vi "Linecut.vi"() -> ()   [LabVIEW 2019]
uses:
  graph_utilities.lvclass
panel:
  out "x-y":dbl
  in  "OK":bool
  in  "width (horizontal) 2":dbl=0.2
  in  "width (vertical) 2":dbl=0.2
  out "Horizontal 2":cluster{dbl[], dbl[]}[](graph)
  out "Vertical 2":cluster{dbl[], dbl[]}[](graph)
  out "Target:":dbl[][](graph)
  in  "width (horizontal)":dbl=0.2
  in  "width (vertical)":dbl=0.2
  out "Horizontal":cluster{dbl[], dbl[]}[](graph)
  out "Vertical":cluster{dbl[], dbl[]}[](graph)
  out "Control:":dbl[][](graph)
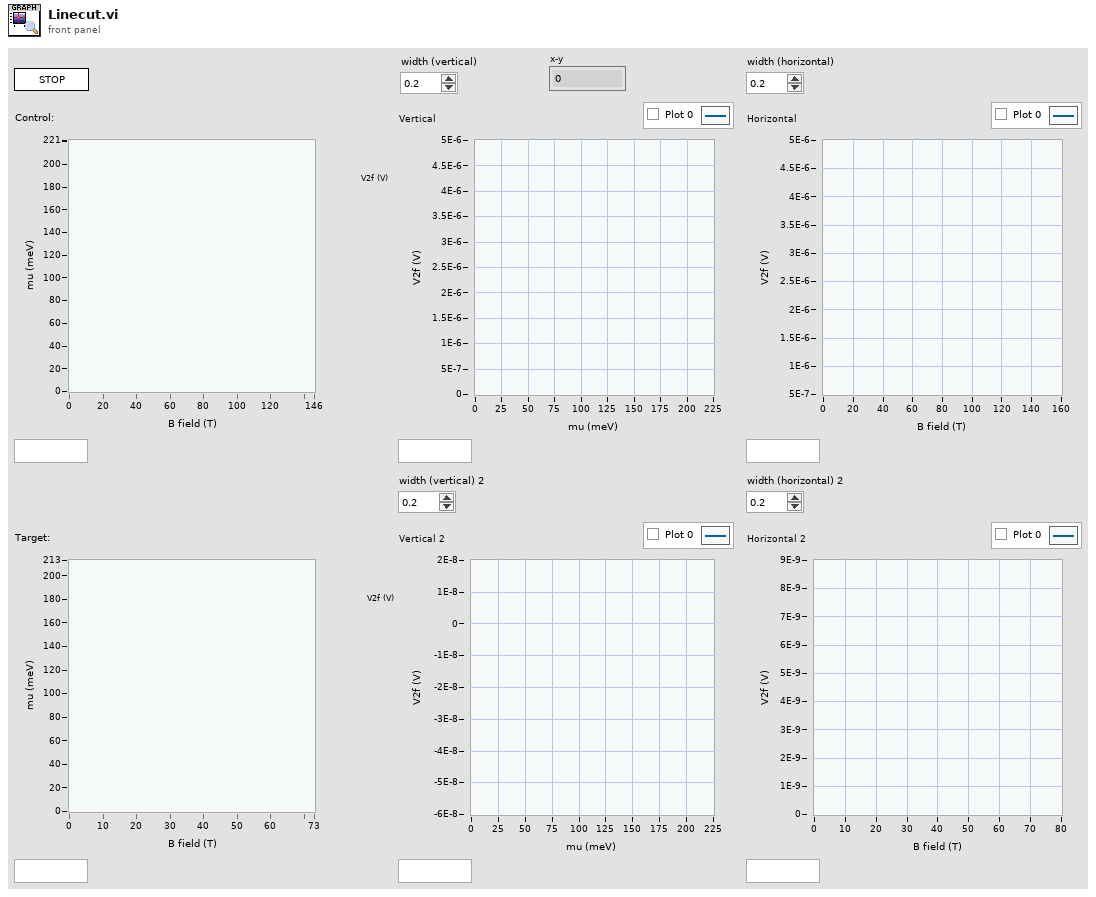
[diagram p1: front panel]
types:
  T1 = enum32{"Invalid", "Standard", "Closed", "Hidden", "Minimized", "Maximized"}
  T2 = enum32{"invalid app kind", "Development System", "Run Time System", "Student Edition", "Embedded LabVIEW", "Evaluation", "Custom"}
  T3 = cluster{"Core":cluster{"Current VI Reference":refnum<vi>, "Close Panel on Exit?":bool}, "graphs":refnum<class "graph_utilities.lvclass">[]}
  T4 = cluster{"Current VI Reference":refnum<vi>, "Close Panel on Exit?":bool}
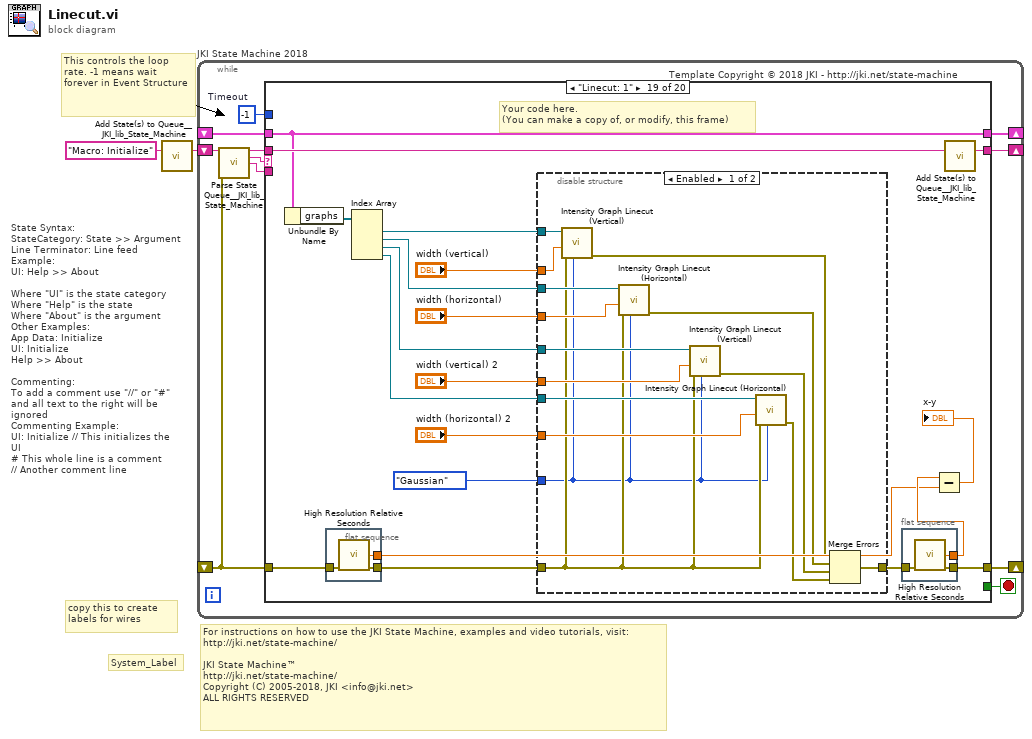
[diagram p0: block diagram]
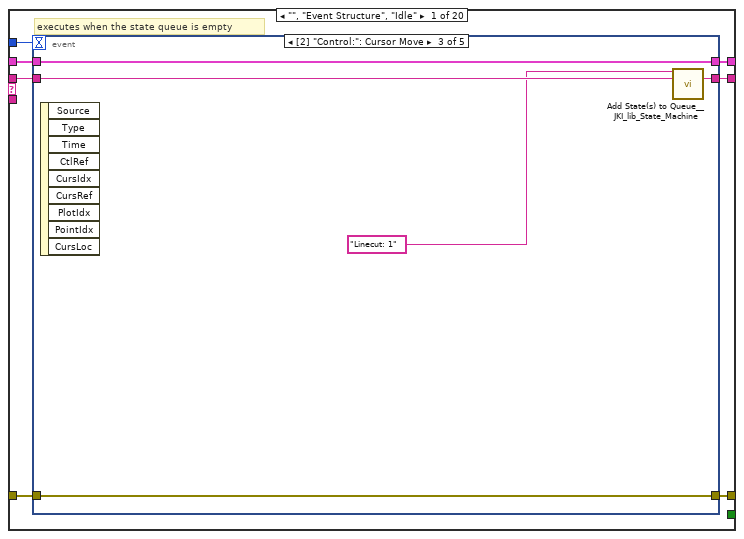
[diagram p2: hidden frame]
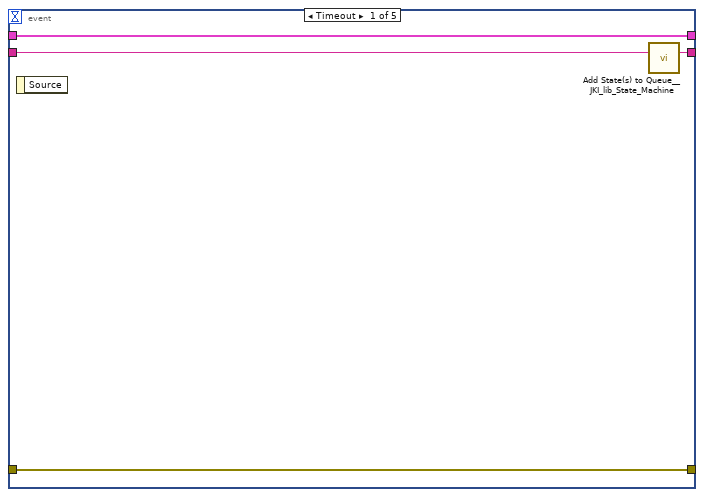
[diagram p3: hidden frame]
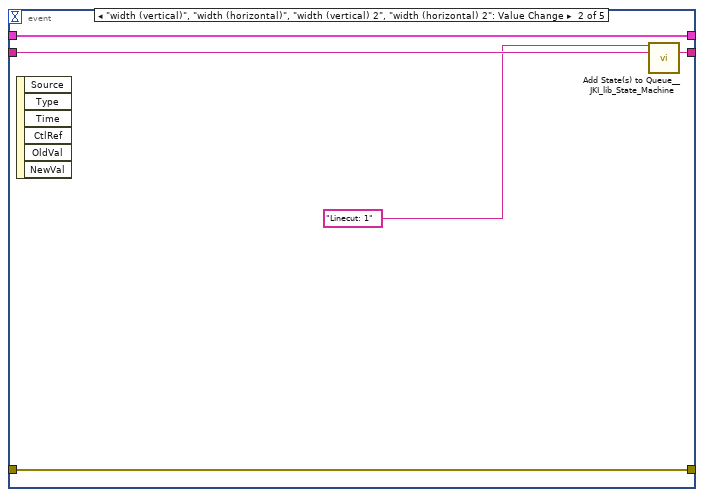
[diagram p4: hidden frame]
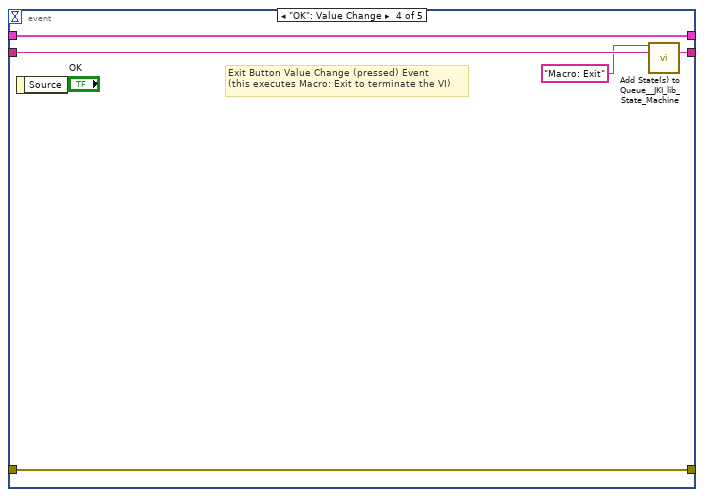
[diagram p5: hidden frame]
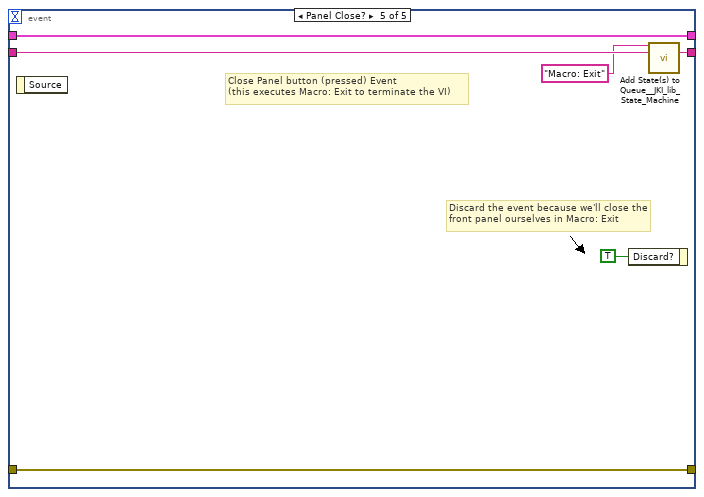
[diagram p6: hidden frame]
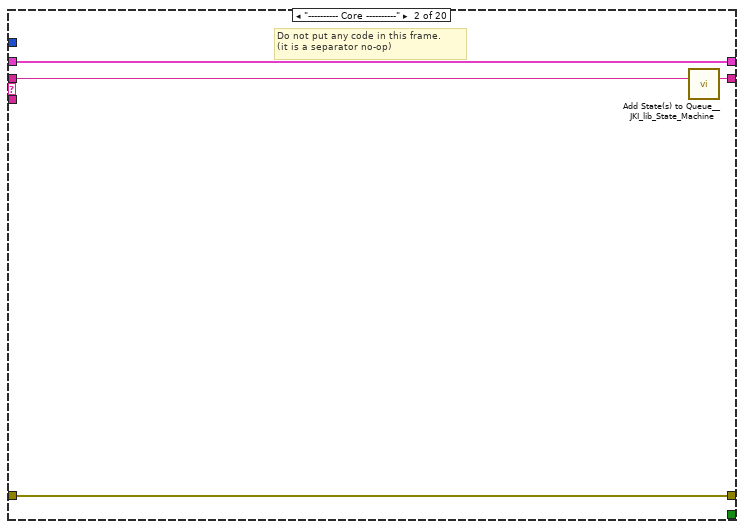
[diagram p7: hidden frame]
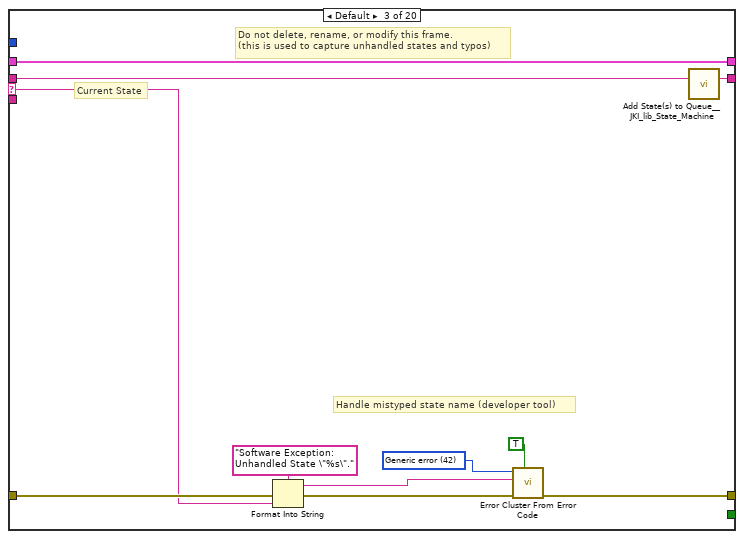
[diagram p8: hidden frame]
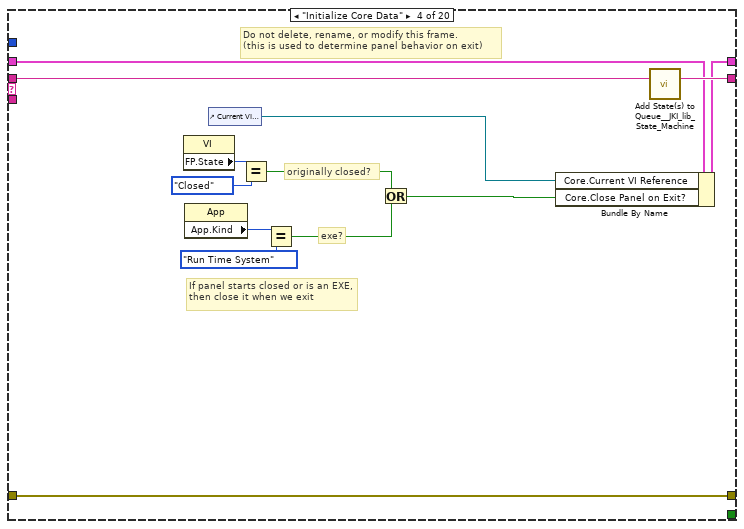
[diagram p9: hidden frame]
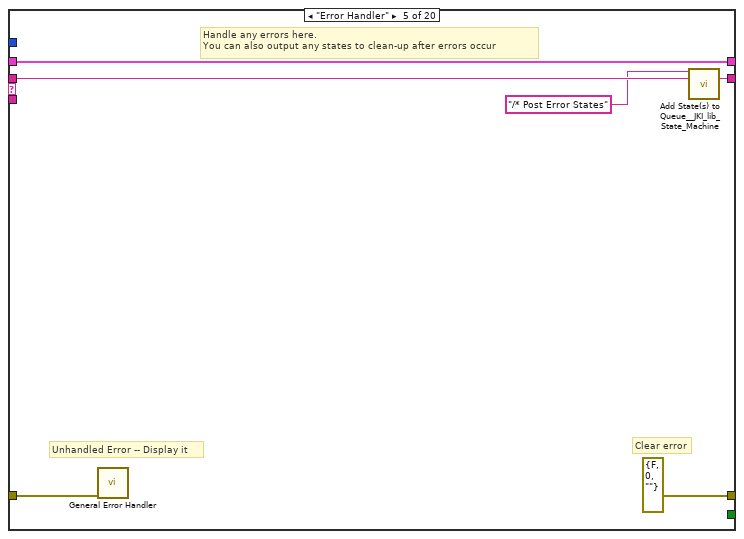
[diagram p10: hidden frame]
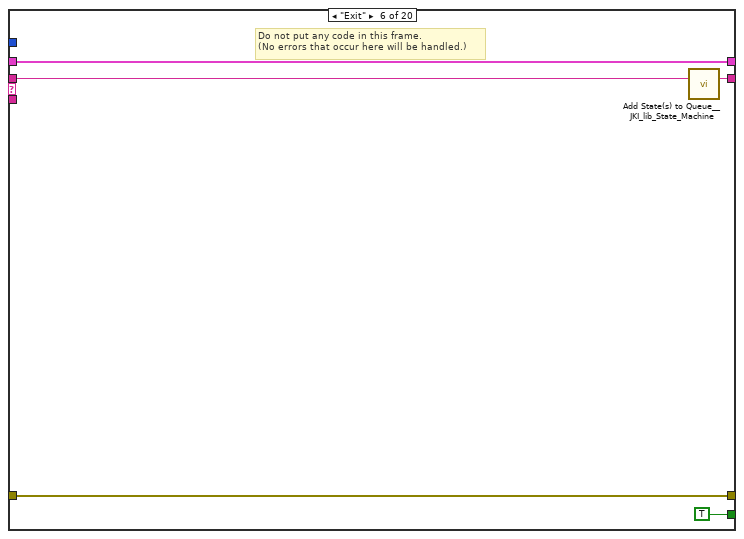
[diagram p11: hidden frame]
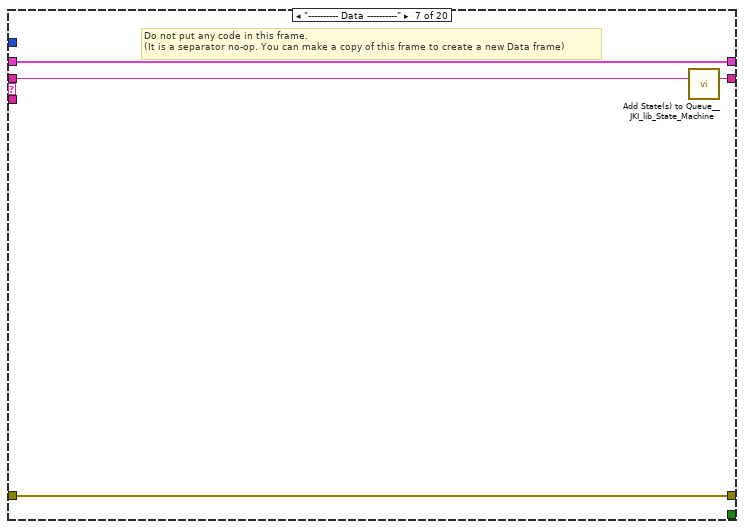
[diagram p12: hidden frame]
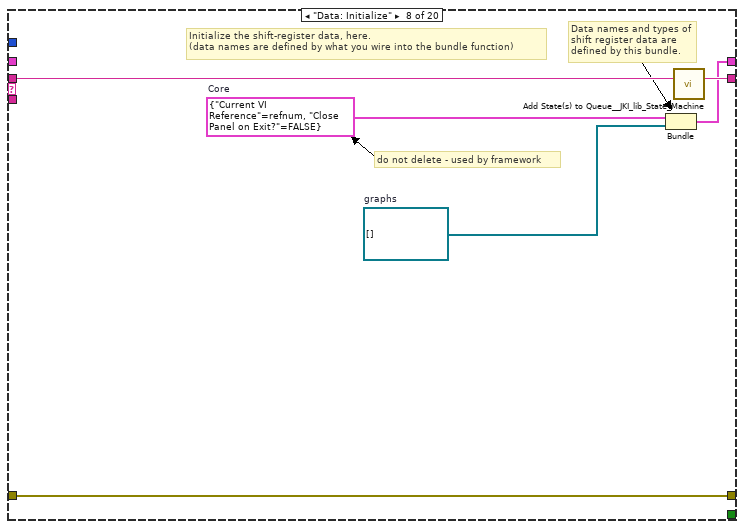
[diagram p13: hidden frame]
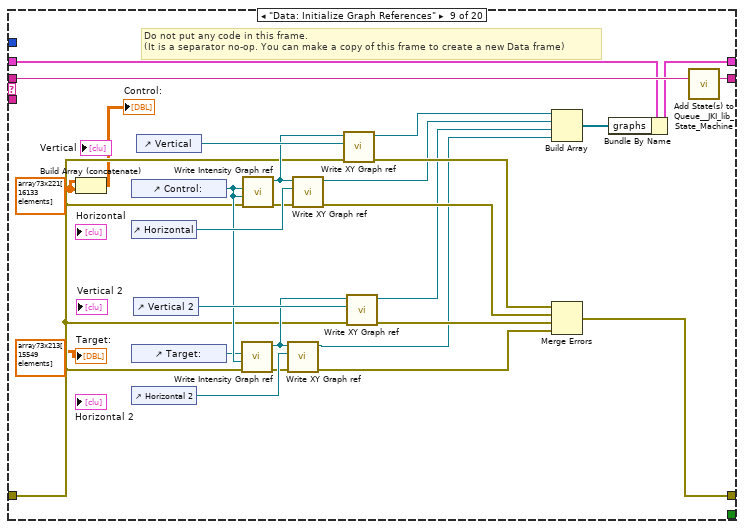
[diagram p14: hidden frame]
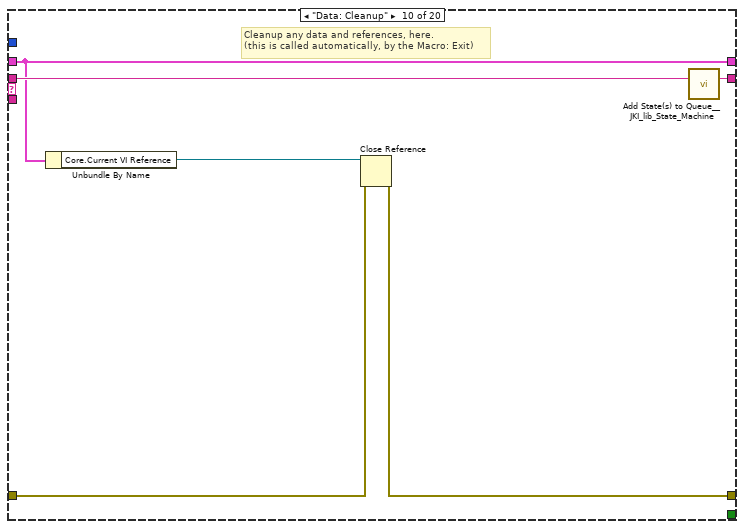
[diagram p15: hidden frame]
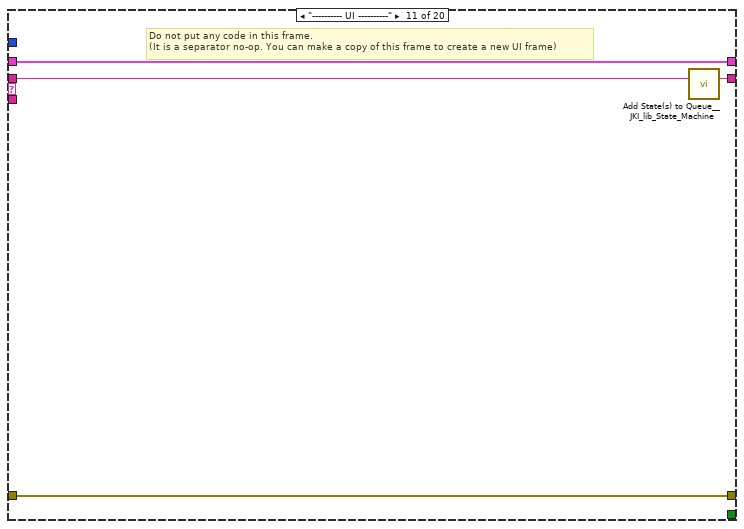
[diagram p16: hidden frame]
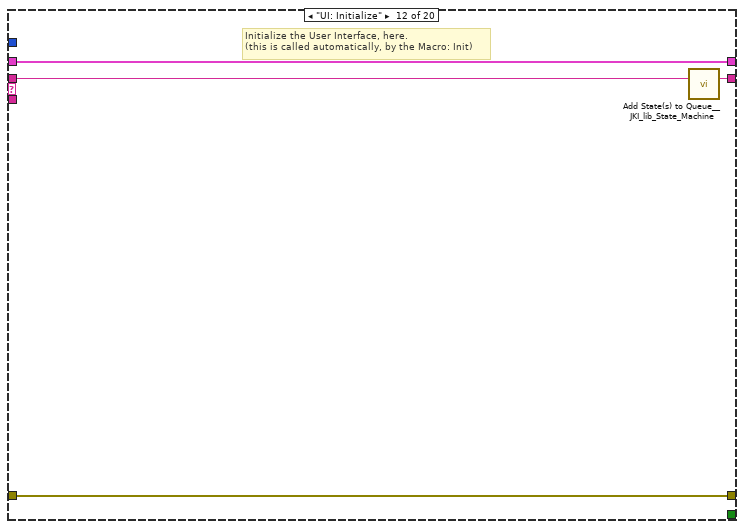
[diagram p17: hidden frame]
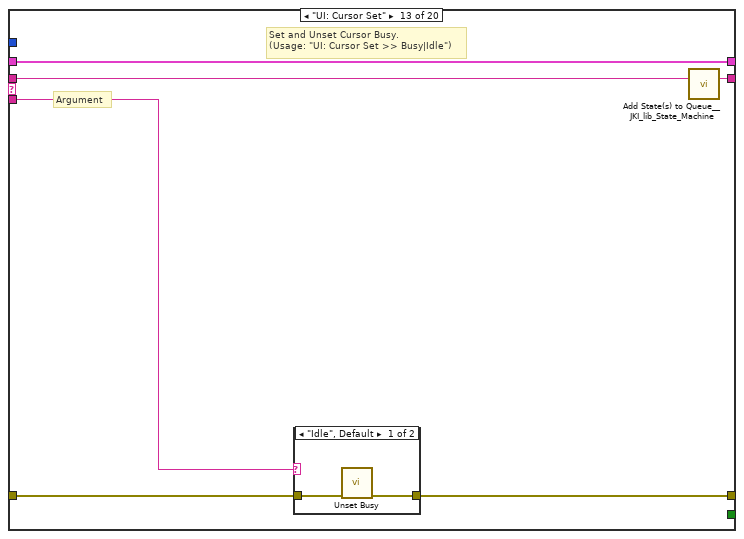
[diagram p18: hidden frame]
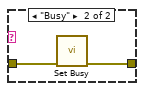
[diagram p19: hidden frame]
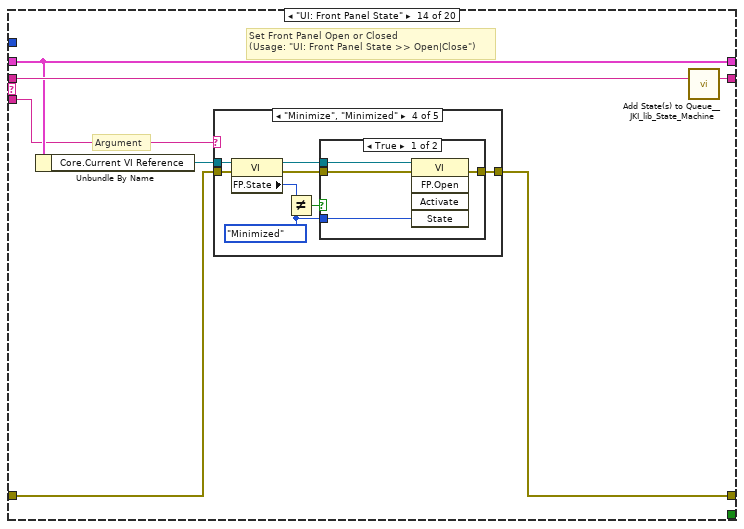
[diagram p20: hidden frame]
diagram:
  # "For instructions on how to use the JKI State Machine, examples and video tutorials, visit:\nhttp://jki.net/state-machine/\n\nJKI State Machine™\nhttp://jki.net/state-machine/\nCopyright (C) 2005-2018, JKI <info@jki.net>\nALL RIGHTS RESERVED"
  # "State Syntax:\nStateCategory: State >> Argument\nLine Terminator: Line feed\nExample:\nUI: Help >> About\n\nWhere \"UI\" is the state category\nWhere \"Help\" is the state\nWhere \"About\" is the argument\nOther Examples:\nApp Data: Initialize\nUI: Initialize\nHelp >> About\n\nCommenting:\nTo add a comment use \"//\" or \"#\" and all text to the right will be ignored\nCommenting Example:\nUI: Initialize // This initializes the UI\n# This whole line is a comment\n// Another comment line"
  # "copy this to create labels for wires"
  # "This controls the loop rate. -1 means wait forever in Event Structure"
  # "System_Label"
  n1 = call <vilib>:"Add State(s) to Queue__JKI_lib_State_Machine.vi"("State(s) in (\"\")"="Macro: Initialize") -> ("States Out"=w2:string)  [unwired: 14 in]
  n2 = while "JKI State Machine 2018" {
    shift-right: [w6] -> _
    shift-left: _ -> [w5]
    shift-right: [w9] -> _
    shift-left: _ -> [w3]
    shift-right: [w8] -> _
    shift-left: w2 -> [w10]
    stop <- w7 stop-if-true
    w4 = -1  # Timeout
    # "Template Copyright © 2018 JKI - http://jki.net/state-machine"
    n3 = call <vilib>:"Parse State Queue__JKI_lib_State_Machine.vi"("State Queue"=w10, "Error In (no error)"=w3) -> ("Remaining States"=w12:string, "Current State"=w13:string, "Arguments"=w11:string)  [unwired: 11 in]
    n4 = case shown="\"Linecut: 1\"" w13 {
      selector: w13 -> [_ _ w50 _ _ _ _ _ _ _ _ _ _ _ _ _ _ _ _ _]
      tunnel: w12 -> [w20 w49 w54 w73 w79 w84 w88 w94 w122 w128 w132 w136 w142 w153 w222 w228 w238 w242 w262 w306]
      tunnel: w11 -> [_ _ _ _ _ _ _ _ _ _ _ _ w137 w147 _ _ _ _ _ _]
      tunnel: w5 -> [w18 w46 w52 w66 w76 w82 w85 _ w106 w123 w129 w134 w140 w149 w219 w225 w235 w239 w257 w303]
      tunnel: [w17 w47 w56 w70 errorcluster {"status"=FALSE, "code"=0, "source"=""} ("error out") w81 w86 w91 w99 w124 w130 w133 w138 w150 w220 w226 w236 w240 w246 w304] -> w9
      tunnel: w3 -> [w16 w47 w55 w70 w75 w81 w86 w91 w98 w125 w130 w133 w139 w151 w220 w226 w236 w240 w249 w304]
      tunnel: [w19 w48 w53 w72 w78 w83 w87 w93 w121 w127 w131 w135 w141 w152 w221 w227 w237 w241 w261 w305] -> w8
      tunnel: [_ _ _ _ _ TRUE _ _ _ _ _ _ _ _ _ _ _ _ _ _] -> w7
      tunnel: [w15 w46 w52 w71 w76 w82 w85 w92 w105 w123 w129 w134 w140 w149 w219 w225 w235 w239 w257 w303] -> w6
      tunnel: w4 -> [w14 _ _ _ _ _ _ _ _ _ _ _ _ _ _ _ _ _ _ _]
      frame "", "Event Structure", "Idle" {
        # "executes when the state queue is empty"
        n5 = event shown="[2] \"Control:\": Cursor Move" {
          selector: _ -> [_ _ _ _ _]
          dyn-events: _ -> [_ _ _ _ _]
          timeout: w14 -> [_ _ _ _ _]
          tunnel: w20 -> [w24 w29 w34 w39 w45]
          tunnel: [w23 w28 w33 w38 w44] -> w19
          tunnel: w18 -> [w21 w26 w31 w36 w42]
          tunnel: [w22 w27 w32 w37 w43] -> w17
          tunnel: w16 -> [w22 w27 w32 w37 w43]
          tunnel: [w21 w26 w31 w36 w42] -> w15
          event Timeout {
            n6 = event-data() -> ()  [unwired: 1 in, 1 out]
            n7 = call <vilib>:"Add State(s) to Queue__JKI_lib_State_Machine.vi"("State(s) in (\"\")"=w24) -> ("States Out"=w23:string)  [unwired: 14 in]
          }
          event "width (vertical)", "width (horizontal)", "width (vertical) 2", "width (horizontal) 2": Value Change {
            n8 = event-data() -> ()  [unwired: 1 in, 6 out]
            n9 = call <vilib>:"Add State(s) to Queue__JKI_lib_State_Machine.vi"("State(s) in Front (\"\")"="Linecut: 1" ("State(s) in Front (\"\")"), "State(s) in (\"\")"=w29) -> ("States Out"=w28:string)  [unwired: 13 in]
          }
          event "Control:": Cursor Move {
            n10 = event-data() -> ()  [unwired: 1 in, 9 out]
            n11 = call <vilib>:"Add State(s) to Queue__JKI_lib_State_Machine.vi"("State(s) in Front (\"\")"="Linecut: 1" ("State(s) in Front (\"\")"), "State(s) in (\"\")"=w34) -> ("States Out"=w33:string)  [unwired: 13 in]
          }
          event "OK": Value Change {
            # "Exit Button Value Change (pressed) Event\n(this executes Macro: Exit to terminate the VI)"
            n12 = event-data() -> ()  [unwired: 1 in, 1 out]
            n13 = call <vilib>:"Add State(s) to Queue__JKI_lib_State_Machine.vi"("State(s) in Front (\"\")"="Macro: Exit", "State(s) in (\"\")"=w39) -> ("States Out"=w38:string)  [unwired: 13 in]
          }
          event Panel Close? {
            # "Discard the event because we'll close the front panel ourselves in Macro: Exit"
            # "Close Panel button (pressed) Event\n(this executes Macro: Exit to terminate the VI)"
            n14 = event-data() -> ()  [unwired: 1 in, 1 out]
            n15 = event-data("Discard?"=TRUE) -> ()  [unwired: 1 in, 1 out]
            n16 = call <vilib>:"Add State(s) to Queue__JKI_lib_State_Machine.vi"("State(s) in Front (\"\")"="Macro: Exit", "State(s) in (\"\")"=w45) -> ("States Out"=w44:string)  [unwired: 13 in]
          }
        }
      }
      frame "---------- Core ----------" {
        # "Do not put any code in this frame.\n(it is a separator no-op)"
        n17 = call <vilib>:"Add State(s) to Queue__JKI_lib_State_Machine.vi"("State(s) in (\"\")"=w49) -> ("States Out"=w48:string)  [unwired: 14 in]
      }
      frame Default {
        w59 = 42 items=["No error", "Argument error", "Memory is full", "Out of zone", "End of file", "File already open", "Generic file I/O error", "File not found", "File permission error", "Disk is full", "Duplicate path", "Too many files open", "System feature not enabled", "Resource file not found", "Cannot add resource", "Resource not found", "Image not found", "Image memory error", "Pen does not exist", "Config type invalid", "Config token not found", "Config parse error", "Config memory error", "Bad external code format", "Bad external code offset", "External code not present", "Null window", "Destroy window error", "Null menu", "Print aborted", "Bad print record", "Print driver error", "Windows error during printing", "Memory error during printing", "Print dialog error", "Generic print error", "Invalid device refnum", "Device not found", "Device parameter error", "Device unit error", "Cannot open device", "Device call aborted", "Generic error", "Cancelled by user", "Object ID too low", "Object ID too high", "Object not in heap", "Unknown heap", "Unknown object (invalid DefProc)", "Unknown object (DefProc not in table)", "Message out of range", "Invalid (null) method", "Unknown message", "Manager call not supported", "Bad address", "Network operation in progress", "Network operation timed out", "Connection is busy", "Network attribute not supported", "Network error", "Address in use", "System out of memory", "Connection aborted", "Connection refused", "Not connected", "Already connected", "Connection closed", "Initialization error (interapplication manager)", "Bad occurrence", "Wait on unbound occurrence handler", "Occurrence queue overflow", "Datalog type conflict", "Unused", "Unrecognized type (interapplication manager)", "Memory corrupt", "Failed to make temporary DLL", "Old CIN version", "Drag socket not found", "Failed to load drop-object", "Failed to register OLE object", "Failed to release OLE object", "Format specifier type mismatch", "Unknown format specifier", "Too few format specifiers", "Too many format specifiers", "Scan failed", "Newer CIN version", "Error converting to variant", "Runtime menu error", "Password tampered", "Variant attribute not found", "Incompatible variant data type", "Event data is not available", "Event Store is not present", "Occurrence is not found", "Event Queue is not created", "Event info is not available", "Refnum passed is NULL", "Error retrieving Class GUID", "Error retrieving CoClass GUID", "Error retrieving TypeLib GUID.", "Bad built application magic bytes.", "Specific driver is different from the specific driver associated with the Logical Name.", "There is no session opened to the class driver.", "Max Error", "MAX - Error with config objects", "MAX - Error loading configuration", "MAX - Group not supported"]
        # "Current State"
        # "Do not delete, rename, or modify this frame.\n(this is used to capture unhandled states and typos)"
        # "Handle mistyped state name (developer tool)"
        n18 = Format Into String(format string="Software Exception: Unhandled State \"%s\"." ("message"), error in=w55, w50) -> (resulting string=w58:string, error out=w57:errorcluster)  [unwired: 1 in]
        n19 = call <vilib>:"Error Cluster From Error Code.vi"("show call chain? (False)"=TRUE, "error in (no error)"=w57, "error message (\"\")"=w58, "error code (0)"=w59) -> ("error out"=w56:errorcluster)  [unwired: 5 in]
        n20 = call <vilib>:"Add State(s) to Queue__JKI_lib_State_Machine.vi"("State(s) in (\"\")"=w54) -> ("States Out"=w53:string)  [unwired: 14 in]
      }
      frame "Initialize Core Data" {
        # "Do not delete, rename, or modify this frame.\n(this is used to determine panel behavior on exit)"
        # "originally closed?"
        # "exe?"
        # "If panel starts closed or is an EXE, then close it when we exit"
        n21 = property class="VI"() -> ("FP.State"=w63:T1)  [unwired: 2 in, 2 out]
        n22 = property class="App"() -> ("App.Kind"=w69:T2)  [unwired: 2 in, 2 out]
        n23 = control-ref of="Current VI Reference"() -> (w64:refnum<vi>)
        n24 = Equal?(x=w63, y=T1."Closed" ("Front Panel Window:State")) -> (x = y?=w61:bool)
        n25 = Equal?(x=w69, y=T2."Run Time System" ("Application:Kind")) -> (x = y?=w67:bool)
        n26 = Or(x=w61, y=w67) -> (x .or. y?=w65:bool)
        n27 = Bundle By Name(cluster=w66, "Core.Current VI Reference"=w64, "Core.Close Panel on Exit?"=w65) -> (w71:T3)
        n28 = call <vilib>:"Add State(s) to Queue__JKI_lib_State_Machine.vi"("State(s) in (\"\")"=w73) -> ("States Out"=w72:string)  [unwired: 14 in]
      }
      frame "Error Handler" {
        # "Unhandled Error -- Display it"
        # "Handle any errors here.\nYou can also output any states to clean-up after errors occur"
        # "Clear error"
        n29 = call <vilib>:"General Error Handler.vi"("error in (no error)"=w75) -> ()  [unwired: 10 in, 5 out]
        n30 = call <vilib>:"Add State(s) to Queue__JKI_lib_State_Machine.vi"("State(s) in Front (\"\")"="/* Post Error States", "State(s) in (\"\")"=w79) -> ("States Out"=w78:string)  [unwired: 13 in]
      }
      frame "Exit" {
        # "Do not put any code in this frame.\n(No errors that occur here will be handled.)"
        n31 = call <vilib>:"Add State(s) to Queue__JKI_lib_State_Machine.vi"("State(s) in (\"\")"=w84) -> ("States Out"=w83:string)  [unwired: 14 in]
      }
      frame "---------- Data ----------" {
        # "Do not put any code in this frame.\n(It is a separator no-op. You can make a copy of this frame to create a new Data frame)"
        n32 = call <vilib>:"Add State(s) to Queue__JKI_lib_State_Machine.vi"("State(s) in (\"\")"=w88) -> ("States Out"=w87:string)  [unwired: 14 in]
      }
      frame "Data: Initialize" {
        w89 = refnum<class "graph_utilities.lvclass">[] []  # graphs
        w90 = T4 {"Current VI Reference"=refnum, "Close Panel on Exit?"=FALSE}  # Core
        # "do not delete - used by framework"
        # "Data names and types of shift register data are defined by this bundle."
        # "Initialize the shift-register data, here.\n(data names are defined by what you wire into the bundle function)"
        n33 = Bundle("Core"=w90, "graphs"=w89) -> (w92:T3)  [unwired: 1 in]
        n34 = call <vilib>:"Add State(s) to Queue__JKI_lib_State_Machine.vi"("State(s) in (\"\")"=w94) -> ("States Out"=w93:string)  [unwired: 14 in]
      }
      frame "Data: Initialize Graph References" {
        w95 = dbl[][] array73x221[16133 elements] ("V2f")
        # "Do not put any code in this frame.\n(It is a separator no-op. You can make a copy of this frame to create a new Data frame)"
        n35 = Build Array (concatenate)(w95, w95) -> (→"Control:":dbl[][])
        n36 = control-ref of="Control:"() -> (w112:refnum<vi>)
        n37 = control-ref of="Horizontal"() -> (w114:refnum<vi>)
        n38 = control-ref of="Target:"() -> (w111:refnum<vi>)
        n39 = control-ref of="Horizontal 2"() -> (w117:refnum<vi>)
        n40 = control-ref of="Vertical 2"() -> (w119:refnum<vi>)
        n41 = control-ref of="Vertical"() -> (w120:refnum<vi>)
        n42 = call "Write Intensity Graph ref.vi"("error in (no error)"=w98, "Intensity Graph (Control)"=w112, "Intensity Graph"=w111) -> ("error out"=w116:errorcluster, "graph_utilities out"=w118:refnum<class "graph_utilities.lvclass">)  [unwired: 7 in]
        n43 = call "Write Intensity Graph ref.vi"("error in (no error)"=w98, "Intensity Graph (Control)"=w112, "Intensity Graph"=w112) -> ("error out"=w113:errorcluster, "graph_utilities out"=w115:refnum<class "graph_utilities.lvclass">)  [unwired: 7 in]
        n44 = call "Write XY Graph ref.vi"("error in (no error)"=w116, "XY Graph"=w117, "graph_utilities in"=w118) -> ("error out"=w110:errorcluster, "graph_utilities out"=w101:refnum<class "graph_utilities.lvclass">)  [unwired: 7 in]
        n45 = call "Write XY Graph ref.vi"("error in (no error)"=w113, "XY Graph"=w114, "graph_utilities in"=w115) -> ("error out"=w108:errorcluster, "graph_utilities out"=w103:refnum<class "graph_utilities.lvclass">)  [unwired: 7 in]
        n46 = call "Write XY Graph ref.vi"("error in (no error)"=w98, "XY Graph"=w120, "graph_utilities in"=w115) -> ("error out"=w107:errorcluster, "graph_utilities out"=w104:refnum<class "graph_utilities.lvclass">)  [unwired: 7 in]
        n47 = call "Write XY Graph ref.vi"("error in (no error)"=w98, "XY Graph"=w119, "graph_utilities in"=w118) -> ("error out"=w109:errorcluster, "graph_utilities out"=w102:refnum<class "graph_utilities.lvclass">)  [unwired: 7 in]
        n48 = Build Array(w104, w103, w102, w101) -> (w100:refnum<class "graph_utilities.lvclass">[])
        n49 = Merge Errors(w107, w108, w109, w110) -> (w99:errorcluster)
        n50 = Bundle By Name(cluster=w106, "graphs"=w100) -> (w105:T3)
        n51 = call <vilib>:"Add State(s) to Queue__JKI_lib_State_Machine.vi"("State(s) in (\"\")"=w122) -> ("States Out"=w121:string)  [unwired: 14 in]
        "Target:" <- dbl[][] array73x213[15549 elements] ("V2f 2")
      }
      frame "Data: Cleanup" {
        # "Cleanup any data and references, here.\n(this is called automatically, by the Macro: Exit)"
        n52 = Unbundle By Name(w123) -> ("Core.Current VI Reference"=w126:refnum<vi>)
        n53 = Close Reference(reference=w126, error in (no error)=w125) -> (error out=w124:errorcluster)
        n54 = call <vilib>:"Add State(s) to Queue__JKI_lib_State_Machine.vi"("State(s) in (\"\")"=w128) -> ("States Out"=w127:string)  [unwired: 14 in]
      }
      frame "---------- UI ----------" {
        # "Do not put any code in this frame.\n(It is a separator no-op. You can make a copy of this frame to create a new UI frame)"
        n55 = call <vilib>:"Add State(s) to Queue__JKI_lib_State_Machine.vi"("State(s) in (\"\")"=w132) -> ("States Out"=w131:string)  [unwired: 14 in]
      }
      frame "UI: Initialize" {
        # "Initialize the User Interface, here.\n(this is called automatically, by the Macro: Init)"
        n56 = call <vilib>:"Add State(s) to Queue__JKI_lib_State_Machine.vi"("State(s) in (\"\")"=w136) -> ("States Out"=w135:string)  [unwired: 14 in]
      }
      frame "UI: Cursor Set" {
        # "Argument"
        # "Set and Unset Cursor Busy.\n(Usage: \"UI: Cursor Set >> Busy|Idle\")"
        n57 = case shown="\"Idle\", Default" w137 {
          tunnel: w139 -> [w144 w146]
          tunnel: [w143 w145] -> w138
          frame "Idle", Default {
            n58 = call <vilib>:"Unset Busy.vi"("error in (no error)"=w144) -> ("error out"=w143:errorcluster)  [unwired: 10 in]
          }
          frame "Busy" {
            n59 = call <vilib>:"Set Busy.vi"("error in (no error)"=w146) -> ("error out"=w145:errorcluster)  [unwired: 9 in, 1 out]
          }
        }
        n60 = call <vilib>:"Add State(s) to Queue__JKI_lib_State_Machine.vi"("State(s) in (\"\")"=w142) -> ("States Out"=w141:string)  [unwired: 14 in]
      }
      frame "UI: Front Panel State" {
        # "Argument"
        # "Set Front Panel Open or Closed\n(Usage: \"UI: Front Panel State >> Open|Close\")"
        n61 = Unbundle By Name(w149) -> ("Core.Current VI Reference"=w148:refnum<vi>)
        n62 = case shown="\"Minimize\", \"Minimized\"" w147 {
          tunnel: w151 -> [w159 w174 w185 w198 w211]
          tunnel: [w161 w175 w187 w200 w213] -> w150
          tunnel: w148 -> [w160 w172 w186 w199 w212]
          frame "Open", "Standard", Default {
            w154 = T1."Standard" ("State")
            n63 = property class="VI"(reference=w160, error in=w159) -> (reference out=w157:refnum<vi>, error out=w158:errorcluster, "FP.State"=w156:T1)
            n64 = Not Equal?(x=w156, y=w154) -> (x != y?=w155:bool)
            n65 = case shown="True" w155 {
              tunnel: [w165 w167] -> w161
              tunnel: w158 -> [w164 w167]
              tunnel: w157 -> [w163 _]
              tunnel: w154 -> [w162 _]
              frame True {
                n66 = invoke class="VI" method="FP.Open"(reference=w163, error in=w164, "Activate"=TRUE, "State"=w162) -> (error out=w165:errorcluster)  [unwired: 1 in, 4 out]
              }
              frame False {
              }
            }
          }
          frame "Close", "Closed" {
            n67 = property class="VI"(reference=w172, error in=w174) -> (reference out=w171:refnum<vi>, error out=w173:errorcluster, "FP.State"=w169:T1)
            n68 = Not Equal?(x=w169, y=T1."Closed" ("Front Panel Window:State")) -> (x != y?=w168:bool)
            n69 = case shown="True" w168 {
              tunnel: [w176 w179] -> w175
              tunnel: w173 -> [w176 w178]
              tunnel: w171 -> [_ w177]
              frame False {
              }
              frame True {
                n70 = invoke class="VI" method="FP.Close"(reference=w177, error in=w178) -> (error out=w179:errorcluster)  [unwired: 1 in, 2 out]
              }
            }
          }
          frame "Hidden", "Hide" {
            w180 = T1."Hidden" ("State")
            n71 = property class="VI"(reference=w186, error in=w185) -> (reference out=w183:refnum<vi>, error out=w184:errorcluster, "FP.State"=w182:T1)
            n72 = Not Equal?(x=w182, y=w180) -> (x != y?=w181:bool)
            n73 = case shown="True" w181 {
              tunnel: [w191 w192] -> w187
              tunnel: w184 -> [w190 w192]
              tunnel: w183 -> [w189 _]
              tunnel: w180 -> [w188 _]
              frame True {
                n74 = invoke class="VI" method="FP.Open"(reference=w189, error in=w190, "State"=w188) -> (error out=w191:errorcluster)  [unwired: 2 in, 4 out]
              }
              frame False {
              }
            }
          }
          frame "Minimize", "Minimized" {
            w193 = T1."Minimized" ("State")
            n75 = property class="VI"(reference=w199, error in=w198) -> (reference out=w196:refnum<vi>, error out=w197:errorcluster, "FP.State"=w195:T1)
            n76 = Not Equal?(x=w195, y=w193) -> (x != y?=w194:bool)
            n77 = case shown="True" w194 {
              tunnel: [w204 w205] -> w200
              tunnel: w197 -> [w203 w205]
              tunnel: w196 -> [w202 _]
              tunnel: w193 -> [w201 _]
              frame True {
                n78 = invoke class="VI" method="FP.Open"(reference=w202, error in=w203, "State"=w201) -> (error out=w204:errorcluster)  [unwired: 2 in, 4 out]
              }
              frame False {
              }
            }
          }
          frame "Maximize", "Maximized" {
            w206 = T1."Maximized" ("State")
            n79 = property class="VI"(reference=w212, error in=w211) -> (reference out=w209:refnum<vi>, error out=w210:errorcluster, "FP.State"=w208:T1)
            n80 = Not Equal?(x=w208, y=w206) -> (x != y?=w207:bool)
            n81 = case shown="True" w207 {
              tunnel: [w217 w218] -> w213
              tunnel: w210 -> [w216 w218]
              tunnel: w209 -> [w215 _]
              tunnel: w206 -> [w214 _]
              frame True {
                n82 = invoke class="VI" method="FP.Open"(reference=w215, error in=w216, "State"=w214) -> (error out=w217:errorcluster)  [unwired: 2 in, 4 out]
              }
              frame False {
              }
            }
          }
        }
        n83 = call <vilib>:"Add State(s) to Queue__JKI_lib_State_Machine.vi"("State(s) in (\"\")"=w153) -> ("States Out"=w152:string)  [unwired: 14 in]
      }
      frame "---------- Macro ----------" {
        # "Do not put any code in this frame.\n(It is a separator no-op. You can make a copy of this frame to create a new Macro frame)"
        n84 = call <vilib>:"Add State(s) to Queue__JKI_lib_State_Machine.vi"("State(s) in (\"\")"=w222) -> ("States Out"=w221:string)  [unwired: 14 in]
      }
      frame "Macro: Initialize" {
        w224 = "Data: Initialize\nInitialize Core Data\nUI: Initialize\nUI: Front Panel State >> Open"  # Data: Initialize Initialize Core Data UI: Initialize UI: Front Panel State >> Open
        # "Initialization Macro\n(This is called once, when the VI starts)"
        n85 = call <vilib>:"Add State(s) to Queue__JKI_lib_State_Machine.vi"("State(s) in Front (\"\")"=w224, "State(s) in (\"\")"=w228, "State(s) at Back (\"\")"="Data: Initialize Graph References\nLinecut: 1") -> ("States Out"=w227:string)  [unwired: 12 in]
      }
      frame "Macro: Exit" {
        # "Exit Macro\n(This is called once, when the VI exits)"
        n86 = Unbundle By Name(w235) -> ("Core.Close Panel on Exit?"=w234:bool)
        n87 = Select(t="UI: Front Panel State >> Close", s=w234, f="") -> (s? t:f=w231:string)
        n88 = call <vilib>:"Add State(s) to Queue__JKI_lib_State_Machine.vi"("State(s) in (\"\")"=w231, "State(s) at Back (\"\")"="Data: Cleanup\nExit") -> ("States Out"=w229:string)  [unwired: 13 in]
        n89 = call <vilib>:"Add State(s) to Queue__JKI_lib_State_Machine.vi"("State(s) in Front (\"\")"=w229, "State(s) in (\"\")"=w238) -> ("States Out"=w237:string)  [unwired: 13 in]
      }
      frame "---------- Linecut ----------" {
        # "Template Separator\n(You can make a copy of, or modify, this frame)"
        n90 = call <vilib>:"Add State(s) to Queue__JKI_lib_State_Machine.vi"("State(s) in (\"\")"=w242) -> ("States Out"=w241:string)  [unwired: 14 in]
      }
      frame "Linecut: 1" {
        # "Your code here.\n(You can make a copy of, or modify, this frame)"
        n91 = Unbundle By Name(w257) -> ("graphs"=w256:refnum<class "graph_utilities.lvclass">[])
        n92 = flat-sequence {
          tunnel: [w266] -> w244
          tunnel: [w265] -> w248
          tunnel: w249 -> [w265]
          frame #0 {
            n93 = call <vilib>:"High Resolution Relative Seconds.vi"() -> ("relative seconds"=w266:dbl)
          }
        }
        n94 = Index Array(array=w256) -> (element #1=w255:refnum<class "graph_utilities.lvclass">, element #2=w254:refnum<class "graph_utilities.lvclass">, element #3=w253:refnum<class "graph_utilities.lvclass">, element #4=w252:refnum<class "graph_utilities.lvclass">)  [unwired: 4 in]
        n95 = disable-structure shown="Enabled" {
          disable-tunnel: "width (vertical) 2" -> [w281 w302]
          disable-tunnel: "width (vertical)" -> [w280 w301]
          disable-tunnel: "width (horizontal) 2" -> [w279 w300]
          disable-tunnel: "width (horizontal)" -> [w278 w299]
          disable-tunnel: w255 -> [w277 w298]
          disable-tunnel: w254 -> [w276 w297]
          disable-tunnel: w253 -> [w275 w296]
          disable-tunnel: w252 -> [w274 w295]
          disable-tunnel: w248 -> [w269 w290]
          disable-tunnel: [w268 w289] -> w247
          disable-tunnel: enum16{"Step", "Gaussian"}."Gaussian" ("Averaging Method") -> [w267 w288]
          frame Enabled {
            n96 = call "Intensity Graph Linecut (Vertical).vi"("Averaging Method"=w267, "error in (no error)"=w269, "width (vertical)"=w280, "graph_utilities in"=w277) -> ("error out"=w273:errorcluster)  [unwired: 6 in, 1 out]
            n97 = call "Intensity Graph Linecut (Horizontal).vi"("Averaging Method"=w267, "error in (no error)"=w269, "width (horizontal)"=w278, "graph_utilities in"=w276) -> ("error out"=w272:errorcluster)  [unwired: 6 in, 1 out]
            n98 = call "Intensity Graph Linecut (Vertical).vi"("Averaging Method"=w267, "error in (no error)"=w269, "width (vertical)"=w281, "graph_utilities in"=w275) -> ("error out"=w271:errorcluster)  [unwired: 6 in, 1 out]
            n99 = call "Intensity Graph Linecut (Horizontal).vi"("Averaging Method"=w267, "error in (no error)"=w269, "width (horizontal)"=w279, "graph_utilities in"=w274) -> ("error out"=w270:errorcluster)  [unwired: 6 in, 1 out]
            n100 = Merge Errors(w273, w272, w271, w270) -> (w268:errorcluster)
          }
          frame Disabled {
            n101 = local read "Target:"() -> (w286:dbl[][])
            n102 = local read "Control:"() -> (w287:dbl[][])
            n103 = call "Intensity Graph Linecut (Vertical) (by val).vi"("Averaging Method"=w288, "error in (no error)"=w290, "width (vertical)"=w301, "2D Data"=w287, "graph_utilities in"=w298) -> ("error out"=w294:errorcluster, "XY-data"=w282:cluster{"X-array":dbl[], "Y-array":dbl[]}[])  [unwired: 4 in, 1 out]
            n104 = call "Intensity Graph Linecut (Horizontal) (by val).vi"("Averaging Method"=w288, "error in (no error)"=w290, "width (horizontal)"=w299, "2D Data"=w287, "graph_utilities in"=w297) -> ("error out"=w293:errorcluster, "XY-data"=w283:cluster{"X-array":dbl[], "Y-array":dbl[]}[])  [unwired: 4 in, 1 out]
            n105 = call "Intensity Graph Linecut (Vertical) (by val).vi"("Averaging Method"=w288, "error in (no error)"=w290, "width (vertical)"=w302, "2D Data"=w286, "graph_utilities in"=w296) -> ("error out"=w292:errorcluster, "XY-data"=w284:cluster{"X-array":dbl[], "Y-array":dbl[]}[])  [unwired: 4 in, 1 out]
            n106 = local write "Vertical"(w282) -> ()
            n107 = local write "Horizontal"(w283) -> ()
            n108 = local write "Vertical 2"(w284) -> ()
            n109 = call "Intensity Graph Linecut (Horizontal) (by val).vi"("Averaging Method"=w288, "error in (no error)"=w290, "width (horizontal)"=w300, "2D Data"=w286, "graph_utilities in"=w295) -> ("error out"=w291:errorcluster, "XY-data"=w285:cluster{"X-array":dbl[], "Y-array":dbl[]}[])  [unwired: 4 in, 1 out]
            n110 = local write "Horizontal 2"(w285) -> ()
            n111 = Merge Errors(w294, w293, w292, w291) -> (w289:errorcluster)
          }
        }
        n112 = flat-sequence {
          tunnel: [w264] -> w245
          tunnel: [w263] -> w246
          tunnel: w247 -> [w263]
          frame #0 {
            n113 = call <vilib>:"High Resolution Relative Seconds.vi"() -> ("relative seconds"=w264:dbl)
          }
        }
        n114 = Subtract(x=w245, y=w244) -> (x-y=→"x-y":dbl)
        n115 = call <vilib>:"Add State(s) to Queue__JKI_lib_State_Machine.vi"("State(s) in (\"\")"=w262) -> ("States Out"=w261:string)  [unwired: 14 in]
      }
      frame "Linecut: 2" {
        # "Your code here.\n(You can make a copy of, or modify, this frame)"
        n116 = call <vilib>:"Add State(s) to Queue__JKI_lib_State_Machine.vi"("State(s) in (\"\")"=w306) -> ("States Out"=w305:string)  [unwired: 14 in]
      }
    }
  }
